vi "open_and_read_word.vi"(8 "error in (no error)":errorcluster, 11 "Word_Doc":path=path "C:/Users/MAJOHN/Inter IKEA Group/Labour Law & Work Environment Course - General/Labour Law/02 Working Material/020 The Swedish Model/01_2_Script.docx") -> (3 "Text":string)   [LabVIEW 2018]
panel:
  out "error out":errorcluster
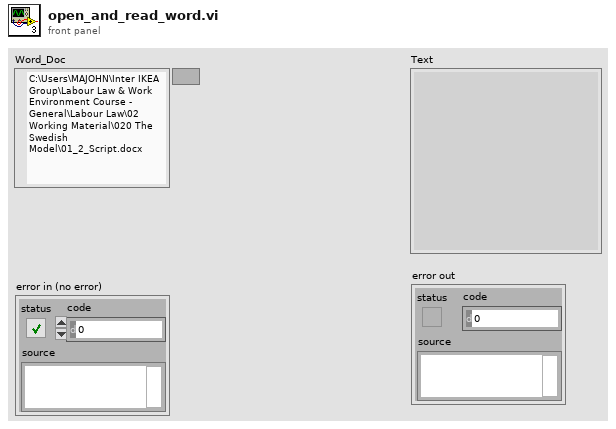
[diagram p1: front panel]
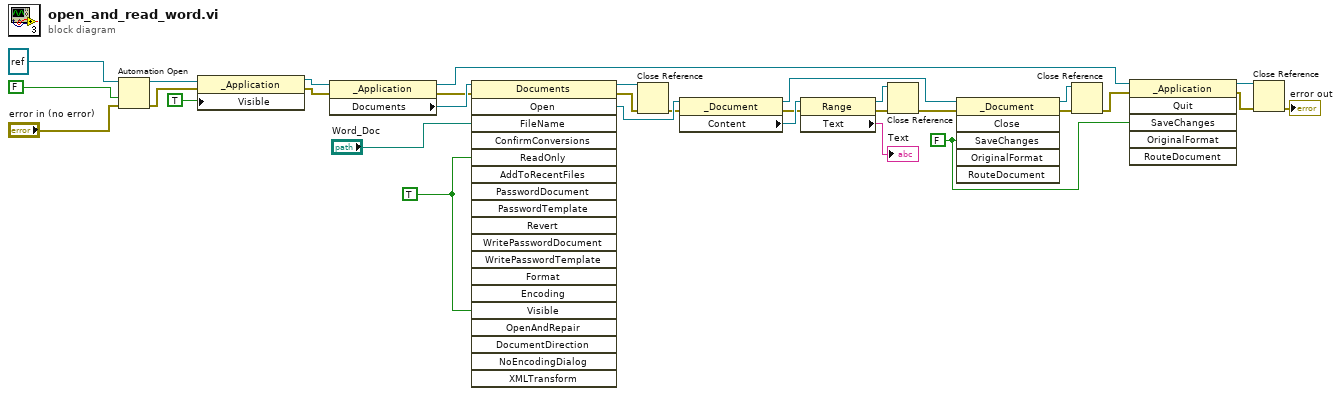
[diagram p0: block diagram]
diagram:
  w18 = FALSE
  w22 = TRUE
  n1 = Automation Open(error in (no error)="error in (no error)", Automation Refnum=refnum<k7> refnum ("Word._Application"), 9:FALSE ("open new instance (false)")) -> (Automation Refnum=w29:refnum<k7>, error out=w27:errorcluster)  [unwired: 1 in]
  n2 = property class="_Application"(reference=w29, error in=w27, "Visible"=TRUE) -> (reference out=w26:refnum<k7>, error out=w25:errorcluster)
  n3 = property class="_Application"(reference=w26, error in=w25) -> (reference out=w19:refnum<k7>, error out=w23:errorcluster, "Documents"=w24:refnum<k7>)
  n4 = invoke class="Documents" method="Open"(reference=w24, error in=w23, "FileName"="Word_Doc", "ReadOnly"=w22, "Visible"=w22) -> (reference out=w14:refnum<k7>, error out=w13:errorcluster, "Open"=w10:refnum<k7>)  [unwired: 14 in, 16 out]
  n5 = Close Reference(reference=w14, error in (no error)=w13) -> (error out=w8:errorcluster)
  n6 = property class="_Document"(reference=w10, error in=w8) -> (reference out=w9:refnum<k7>, error out=w6:errorcluster, "Content"=w12:refnum<k7>)
  n7 = property class="Range"(reference=w12, error in=w6) -> (reference out=w7:refnum<k7>, error out=w5:errorcluster, "Text"=→"Text":string)
  n8 = Close Reference(reference=w7, error in (no error)=w5) -> (error out=w4:errorcluster)
  n9 = invoke class="_Document" method="Close"(reference=w9, error in=w4, "SaveChanges"=w18) -> (reference out=w21:refnum<k7>, error out=w20:errorcluster)  [unwired: 3 in, 4 out]
  n10 = Close Reference(reference=w21, error in (no error)=w20) -> (error out=w3:errorcluster)
  n11 = invoke class="_Application" method="Quit"(reference=w19, error in=w3, "SaveChanges"=w18) -> (reference out=w17:refnum<k7>, error out=w16:errorcluster)  [unwired: 3 in, 4 out]
  n12 = Close Reference(reference=w17, error in (no error)=w16) -> (error out=→"error out":errorcluster)
